vi "Load App.vi"(8 "error in (no error)":errorcluster, 11 "SubProcess in":refnum<class "SubProcess.lvclass">) -> (0 "error out":errorcluster, 3 "SubProcess out":refnum<class "SubProcess.lvclass">)   [LabVIEW 2021, in "SubProcess.lvlib" / "SubProcess.lvclass"]
uses:
  SubProcess.lvclass
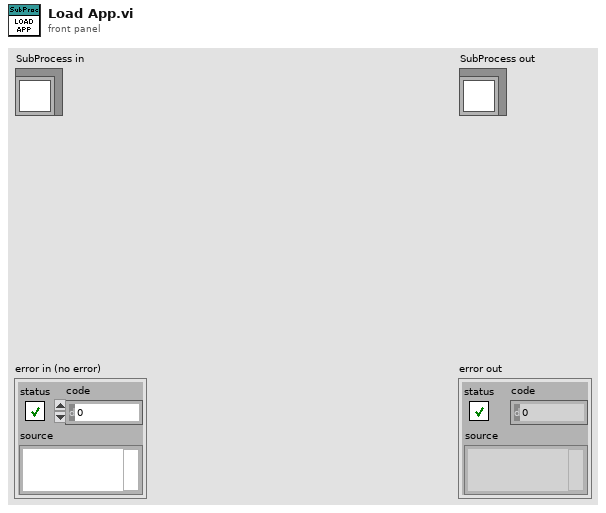
[diagram p1: front panel]
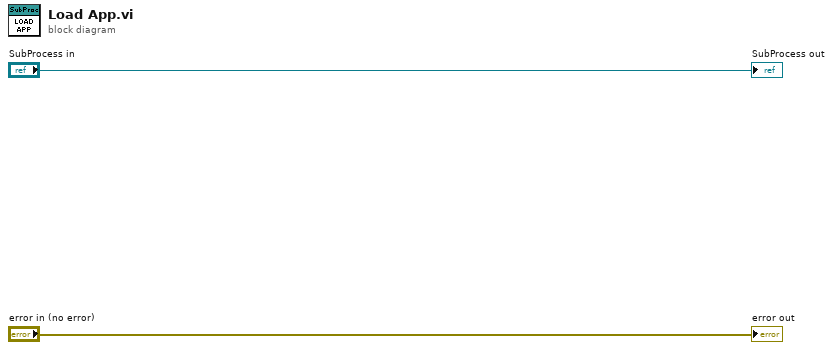
[diagram p0: block diagram]
diagram:
  "error out" <- "error in (no error)"
  "SubProcess out" <- "SubProcess in"
